vi "1_Datalog write.vi"() -> ()   [LabVIEW 2010]
panel:
  out "?":dbl[][](graph)
  in  "Cluster":cluster{"Array":dbl[][]}
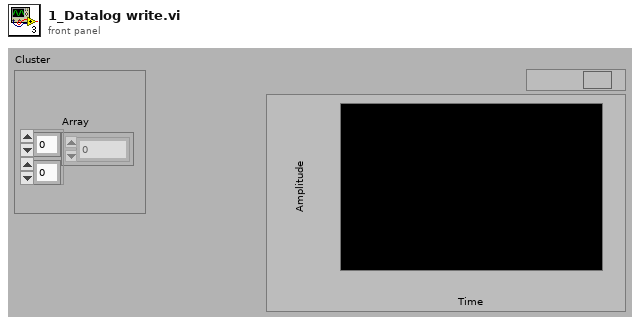
[diagram p1: front panel]
types:
  T1 = enum16{"open", "replace", "create", "open or create", "replace or create", "replace or create with confirmation"}
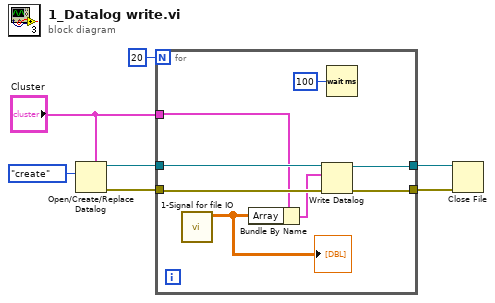
[diagram p0: block diagram]
diagram:
  n1 = Open/Create/Replace Datalog(5:"Cluster", 10:T1."create" ("operation (0:open)")) -> (0:w5:errorcluster, 3:w6:refnum<k1>)  [unwired: 4 in, 1 out]
  n2 = for {
    N: 20 -> [_]
    tunnel: w6 -> [w15]
    tunnel: w5 -> [w12]
    tunnel: [w13] -> w4
    tunnel: [w14] -> w3
    tunnel: "Cluster" -> [w11]
    n3 = call "1-Signal for file IO.vi"() -> ("Data"=w9:dbl[][])  [unwired: 10 in]
    "?" <- w9
    n4 = Bundle By Name(cluster=w11, "Array"=w9) -> (w10:cluster{"Array":dbl[][]})
    n5 = Write Datalog(4:w12, 6:w10, 7:w15) -> (0:w13:errorcluster, 3:w14:refnum<k1>)
    n6 = Wait (ms)(milliseconds to wait=u32 100) -> ()  [unwired: 1 out]
  }
  n7 = Close File(refnum=w3, error in=w4) -> ()  [unwired: 2 out]
